vi "Pad Message String.vi"(1 "Message In":string) -> (0 "Padded Message Out":string)   [LabVIEW 2020, in "Encryption.lvlib"]
uses:
  Encryption.lvlib
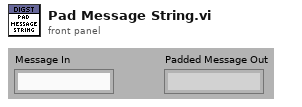
[diagram p1: front panel]
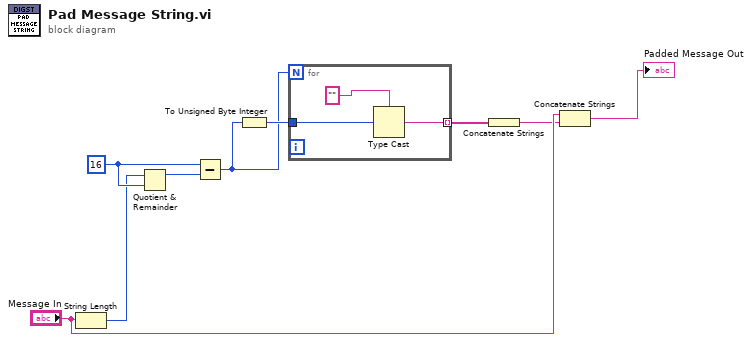
[diagram p0: block diagram]
diagram:
  w2 = 16 ("y")
  n1 = String Length(string="Message In") -> (length=w1:i32)
  n2 = Quotient & Remainder(x=w1, y=w2) -> (x-y*floor(x/y)=w8:i32)  [unwired: 1 out]
  n3 = Subtract(x=w2, y=w8) -> (x-y=w3:i32)
  n4 = To Unsigned Byte Integer(number=w3) -> (unsigned 8bit integer=w4:u8)
  n5 = for {
    N: w3 -> [_]
    tunnel: w4 -> [w12]
    tunnel: [w10] -> w5 mode=indexing
    n6 = Type Cast(type="", x=w12) -> (*(type *) &x=w10:string)
  }
  n7 = Concatenate Strings(w5) -> (w6:string)
  n8 = Concatenate Strings("Message In", w6) -> (→"Padded Message Out":string)
